vi "String Search And Replace.vi"(7 "replace with":string="C", 8 "search for":string="c", 9 "string in":string="abc\n") -> (2 "found":i32=-1, 3 "string out":string)   [LabVIEW 2020]
doc: "This function searches a string for a substring and replaces all occurences of the substring with a new substring."
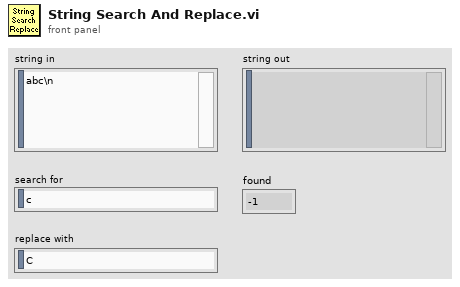
[diagram p1: front panel]
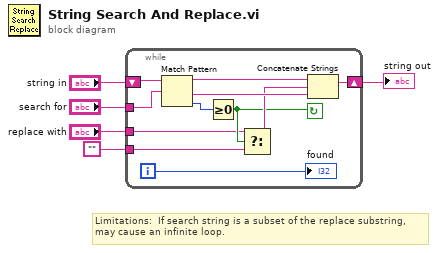
[diagram p0: block diagram]
diagram:
  # "Limitations:  If search string is a subset of the replace substring,\nmay cause an infinite loop."
  n1 = while {
    shift-right: [w9] -> w5
    shift-left: "string in" -> [w11]
    tunnel: "search for" -> [w10]
    tunnel: "replace with" -> [w8]
    tunnel: "" -> [w7]
    i -> [w6]
    stop <- w12 continue-if-true
    n2 = Match Pattern(string=w11, regular expression=w10) -> (before substring=w16:string, after substring=w14:string, offset past match=w15:i32)  [unwired: 1 in, 1 out]
    n3 = Greater Or Equal To 0?(x=w15) -> (x >= 0?=w12:bool)
    n4 = Select(t=w8, s=w12, f=w7) -> (s? t:f=w13:string)
    n5 = Concatenate Strings(w16, w13, w14) -> (w9:string)
    "found" <- w6
  }
  "string out" <- w5
